vi "SetCameraSettings.vi"(2 "error in":errorcluster, 3 "Settings":T2={"Color format"=2, "Hue"=50.0, "Sat"=50.0, "Bright"=50.0, "Contr"=50.0, "Sharp"=50.0, "Black l."=50.0, "White l."=50.0, "Options"=0, "Dialogs"=0} {"Color format" items=["Black & White (8 bits)", "RGB (24 bits)", "RGBx (32 bits)", "RGBA (32bits)", "RGB B&W (32 bits)", "HSI (24 bits)", "HSIx (32 bits)", "HSI B&W (32 bits)"]; "White l." scale=0.0..100.0; "Black l." scale=0.0..100.0; "Sharp" scale=0.0..100.0; "Contr" scale=0.0..100.0; "Bright" scale=0.0..100.0; "Sat" scale=0.0..100.0; "Hue" scale=0.0..100.0}, 4 "QT Ref In":T1) -> (0 "error out":errorcluster, 1 "QT Ref Out":T1)   [LabVIEW 2010]
uses:
  <userlib>/ImageProcessing/CameraSettings.ctl
  <userlib>/ImageProcessing/QTLIB_2595_LV86/QT_Ref.ctl
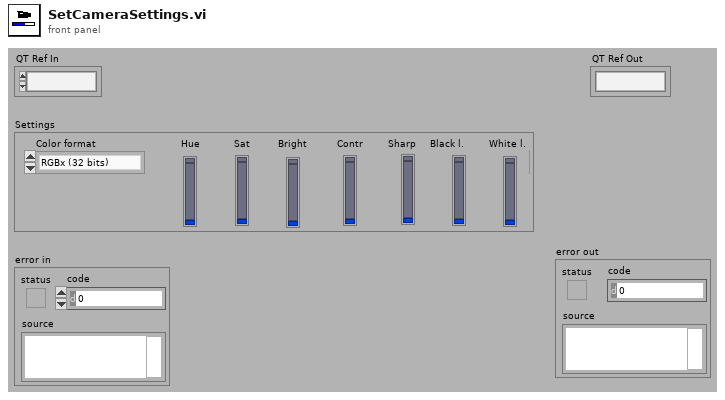
[diagram p1: front panel]
types:
  T1 = typedef "QT_Ref.ctl" = refnum<k1>
  T2 = typedef "CameraSettings.ctl" = cluster{"Color format":u32, "Hue":dbl, "Sat":dbl, "Bright":dbl, "Contr":dbl, "Sharp":dbl, "Black l.":dbl, "White l.":dbl, "Options":i32, "Dialogs":u32}
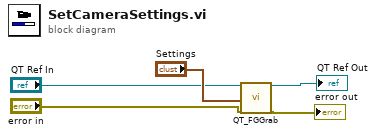
[diagram p0: block diagram]
diagram:
  n1 = call <userlib>:"QT_FGGrab.vi"("QT Ref In"="QT Ref In", "Video Settings in"="Settings", "error in (no error)"="error in") -> ("QT Ref Out"=→"QT Ref Out":T1, "error out"=→"error out":errorcluster)  [unwired: 3 in, 12 out]
